vi "Abort.vi"(1 "Sensor Deadband":dbl, 2 "Sensor":dbl, 3 "Motor Deadband":dbl, 4 "Motor":dbl) -> (0 "Abort":bool)   [LabVIEW 2014]
uses:
  <vilib>/Rock Robotics/WPI/DriverStation/WPI_DriverStationRobotMode2.ctl
  Support Code/Robot Global Data.vi
  <vilib>/addons/control/pid/pid.llb/PID Control Input Filter (DBL).vi
  <vilib>/ptbypt/NI_PtbyPt.lvlib
  <vilib>/addons/control/pid/NI_PID_pid.lvlib
panel:
  out "Waveform Chart":cluster{"Motor Deadband":dbl, "dx/dt":dbl}(graph)
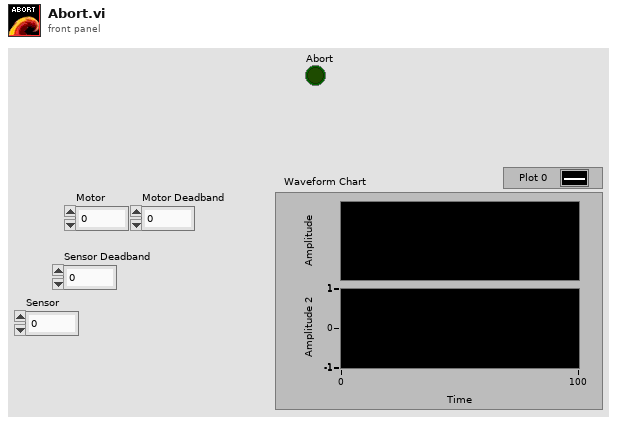
[diagram p1: front panel]
types:
  T1 = typedef "WPI_DriverStationRobotMode2.ctl" = enum16{"Autonomous Disabled", "Autonomous Enabled", "Teleop Disabled", "Teleop Enabled", "Disconnected", "Finish", "Test Disabled", "Test Enabled", "Emergency Stopped"}
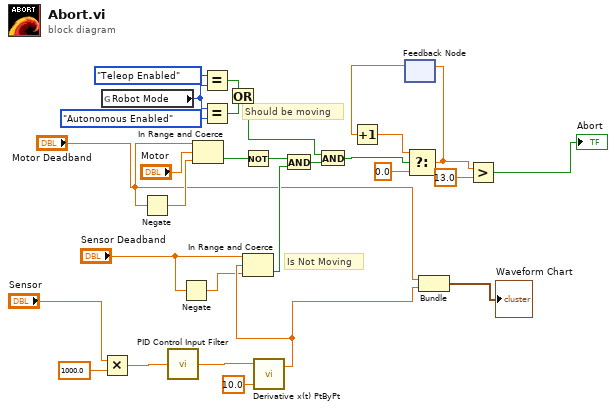
[diagram p0: block diagram]
diagram:
  # "Is Not Moving"
  # "Should be moving"
  n1 = global read "Robot Global Data.vi" "Robot Mode"() -> (w7:T1)
  n2 = Multiply(x="Sensor", y=1000.0) -> (x*y=w19:dbl)
  n3 = Negate(x="Motor Deadband") -> (-x=w28:dbl)
  n4 = call-poly <vilib>:"PID Control Input Filter.vi"("input"=w19) -> ("output"=w18:dbl)  [unwired: 4 in]
  n5 = Negate(x="Sensor Deadband") -> (-x=w15:dbl)
  n6 = In Range and Coerce(upper limit="Motor Deadband", x="Motor", lower limit=w28) -> (In Range?=w27:bool)  [unwired: 1 out]
  n7 = Equal?(x=WPI_DriverStationRobotMode2."Teleop Enabled", y=w7) -> (x = y?=w3:bool)
  n8 = Equal?(x=w7, y=WPI_DriverStationRobotMode2."Autonomous Enabled") -> (x = y?=w4:bool)
  n9 = Or(x=w3, y=w4) -> (x .or. y?=w2:bool)
  n10 = Not(x=w27) -> (.not. x?=w25:bool)
  n11 = call <vilib>:"Derivative x(t) PtByPt.vi"("dt"=10.0, "x"=w18) -> ("dx/dt"=w17:dbl)  [unwired: 2 in, 1 out]
  n12 = In Range and Coerce(upper limit="Sensor Deadband", x=w17, lower limit=w15) -> (In Range?=w26:bool)  [unwired: 1 out]
  n13 = And(x=w25, y=w26) -> (x .and. y?=w8:bool)
  n14 = And(x=w2, y=w8) -> (x .and. y?=w1:bool)
  n15 = feedback #1() -> (w13:dbl)  [unwired: 1 in]
  n16 = Increment(x=w13) -> (x+1=w14:dbl)
  n17 = Select(t=w14, s=w1, f=0.0) -> (s? t:f=w11:dbl)
  n18 = feedback-in #1(w11) -> ()
  n19 = Bundle("Motor Deadband"="Motor Deadband", "dx/dt"=w17) -> (→"Waveform Chart":cluster{"Motor Deadband":dbl, "dx/dt":dbl})  [unwired: 1 in]
  n20 = Greater?(x=w11, y=13.0) -> (0:→"Abort":bool)
